vi "Send Device Meta Data.vi"(8 "error in":errorcluster, 11 "Plugin_Controller in":refnum<class "Plugin_Controller.lvclass">) -> (0 "error out":errorcluster, 3 "Plugin_Controller out":refnum<class "Plugin_Controller.lvclass">)   [LabVIEW 2020, in "Plugin.lvlib" / "Plugin_Controller.lvclass"]
doc: "Send Meta Data details to Node Meta Data Distributor."
uses:
  Plugin_Controller.lvclass
  C:/SVN_LabSys/labsys_lvcode/LabSys_SourceCode/builds/Libraries/LabSys Framework.lvlibp/Data Node/Data Node/Data Node.lvclass
  C:/SVN_LabSys/labsys_lvcode/LabSys_SourceCode/builds/Libraries/LabSys Framework.lvlibp/Devices/Device Driver.lvclass
  builds/Libraries/LabSys Framework.lvlibp/Data Node/Data Node/Read Node Meta Data Distributor.vi
  builds/Libraries/LabSys Framework.lvlibp/Data Node/Data Node/Read Module Name.vi
  builds/Libraries/LabSys Framework.lvlibp/Data Node/Data Node/Write Node Meta Data Distributor.vi
  builds/Libraries/LabSys Framework.lvlibp/Node Meta Data Distributor/Node Meta Data Distributor/Node Meta Data Distributor.lvclass
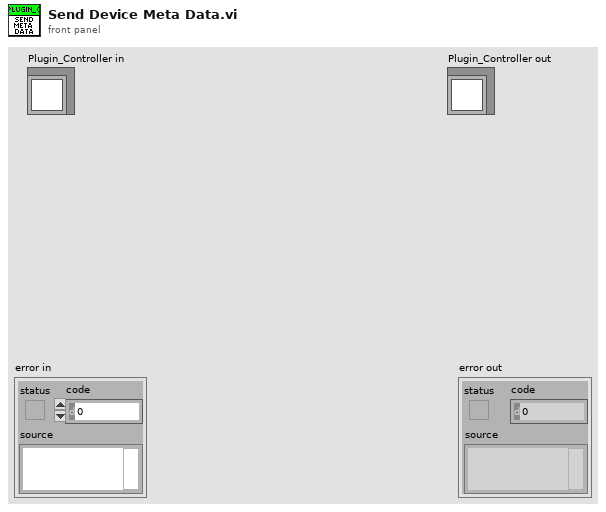
[diagram p1: front panel]
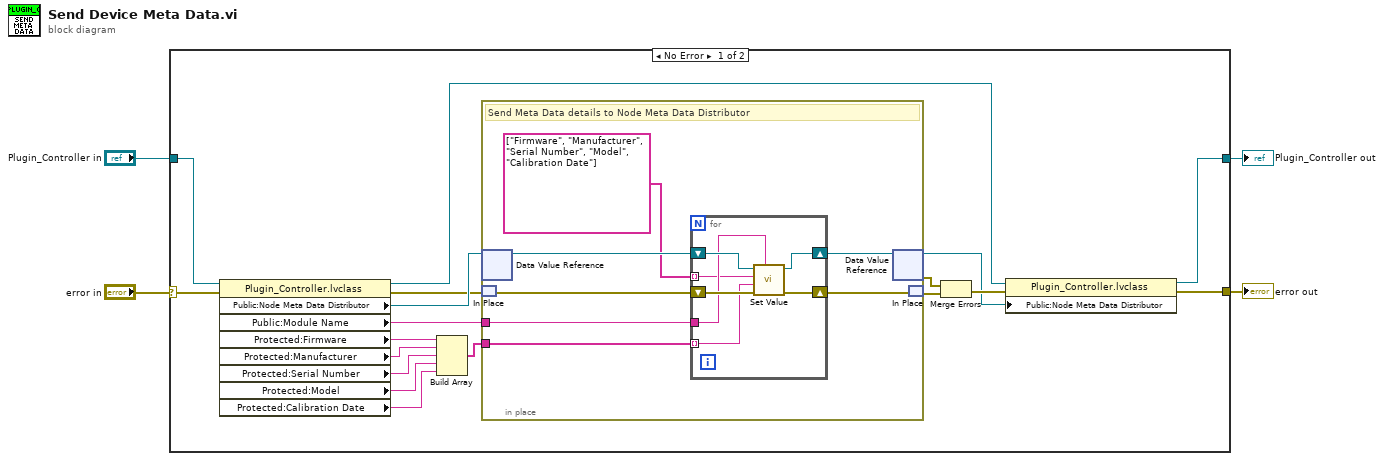
[diagram p0: block diagram]
diagram:
  n1 = case shown="No Error" "error in" {
    selector: "error in" -> [w22 w38]
    tunnel: [w12 w38] -> w4
    tunnel: [w9 w37] -> w1
    tunnel: "Plugin_Controller in" -> [w21 w37]
    frame No Error {
      n2 = property on="Property Node" class="Plugin_Controller.lvclass"(reference=w21, error in=w22) -> (reference out=w10:refnum<class "Plugin_Controller.lvclass">, error out=w19:errorcluster, "Public:Node Meta Data Distributor"=w20:refnum<data-value>, "Public:Module Name"=w18:string, "Protected:Firmware"=w16:string, "Protected:Manufacturer"=w17:string, "Protected:Serial Number"=w7:string, "Protected:Model"=w6:string, "Protected:Calibration Date"=w5:string)
      n3 = Build Array(w16, w17, w7, w6, w5) -> (w15:string[])
      n4 = in-place "In Place Element Structure" {
        in-place-border: w18 -> [w25]
        in-place-border: w15 -> [w24]
        # "Send Meta Data details to Node Meta Data Distributor"
        n5 = in-place-dvr #1(w20) -> (w29:refnum<class "Node Meta Data Distributor.lvclass">)  [unwired: 1 out]
        n6 = in-place-match #2(w19) -> (w28:errorcluster)
        n7 = for {
          tunnel: w25 -> [w32]
          shift-right: [w33] -> w26
          shift-left: w29 -> [w36]
          shift-right: [w34] -> w27
          shift-left: w28 -> [w35]
          tunnel: w24 -> [w31] mode=indexing
          tunnel: string[] ["Firmware", "Manufacturer", "Serial Number", "Model", "Calibration Date"] -> [w30] mode=indexing
          n8 = call "Set Value.vi"("Module Name"=w32, "error in (no error)"=w35, "Value"=w31, "Key"=w30, "Node Meta Data Distributor in"=w36) -> ("error out"=w34:errorcluster, "Node Meta Data Distributor out"=w33:refnum<class "Node Meta Data Distributor.lvclass">)  [unwired: 5 in]
        }
        n9 = in-place-dvr #1(w26) -> (w8:refnum<data-value>, w13:errorcluster)
        n10 = in-place-match #2(w27) -> (w14:errorcluster)
      }
      n11 = Merge Errors(w13, w14) -> (w11:errorcluster)
      n12 = property on="Property Node" class="Plugin_Controller.lvclass"(reference=w10, error in=w11, "Public:Node Meta Data Distributor"=w8) -> (reference out=w9:refnum<class "Plugin_Controller.lvclass">, error out=w12:errorcluster)
    }
    frame Error {
    }
  }
  "error out" <- w4
  "Plugin_Controller out" <- w1
